vi "SANM_FreqMod_Host.vi"() -> ()   [LabVIEW 2012]
uses:
  <vilib>/FPGAPlugInAG/PCI-7831R/niLvFpga_Open_PCI-7831R.vi
  <vilib>/Utility/error.llb/Error Cluster From Error Code.vi
  <vilib>/rvi/errors/niLvFpgaAdjustHostInterfaceError.vi
  <vilib>/FPGAPlugInAG/PCI-7831R/niLvFpga_Abort_PCI-7831R.vi
  <vilib>/FPGAPlugInAG/PCI-7831R/niLvFpga_Close_PCI-7831R.vi
  <vilib>/rvi/interface/nirviOpenFPGA/nirviOpenFPGA.xnode
  SB130-XPS/Documents/FPGA-project-apporach-retraction/FPGA Bitfiles/Apporach-Retract_FPGATarget2_SANMFreqMod-1a_mUEf4QzcPK8.lvbitx
  SANM_FreqMod-1a.vi
  <vilib>/rvi/interface/nirviReadWriteControl/nirviReadWriteControl.xnode
  <vilib>/rvi/interface/nirviMethod/nirviMethod.xnode
  <vilib>/rvi/interface/nirviCloseFPGA/nirviCloseFPGA.xnode
  NiFpgaLv.dll
panel:
  in  "millisecond multiple":u32=75
  out "Indicator":dbl=0.15
  in  "Sampling Frequency 2":i32=200000
  in  "PLL Input\nNominal \nFrequency":i32=30000
  out "R Graph":dbl(graph)
  out "Degree":dbl
  out "Y":dbl
  out "X":dbl
  out "F Graph":dbl(graph)
  in  "Sampling Frequency":dbl=200000.0
  out "Decimation":i32=977
  out "Stages":i32=1
  out "Dec2":i32=128
  out "Dec1":i32=1
  in  "Filter Rolloff":enum16{"20 dB", "40 dB", "60 dB", "80 dB"}(ring)
  in  "Time Constant [s]":dbl=2.5 min=0.0 step=0.0001 format="%.2f"
  in  "stop 2":bool
  in  "stop":bool
  out "K Indicator":dbl=1.52588e-05
  out "Nominal Freq Indicator":dbl=0.494873
  in  "K":dbl=1.52588e-05
  in  "Nominal Freq":dbl=0.494873
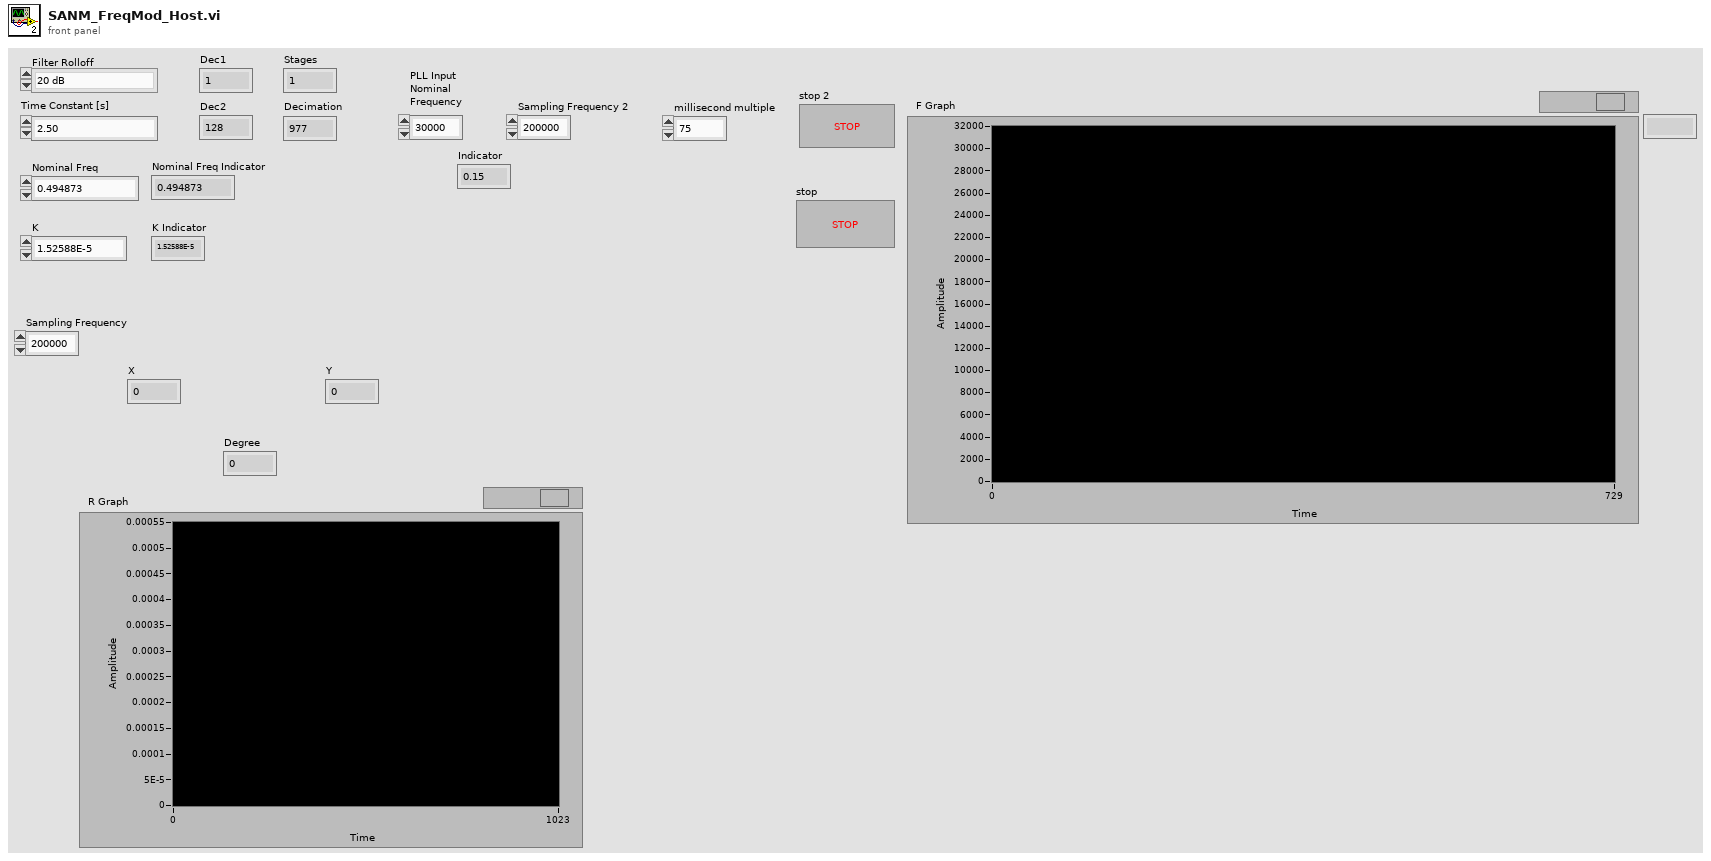
[diagram p1: front panel]
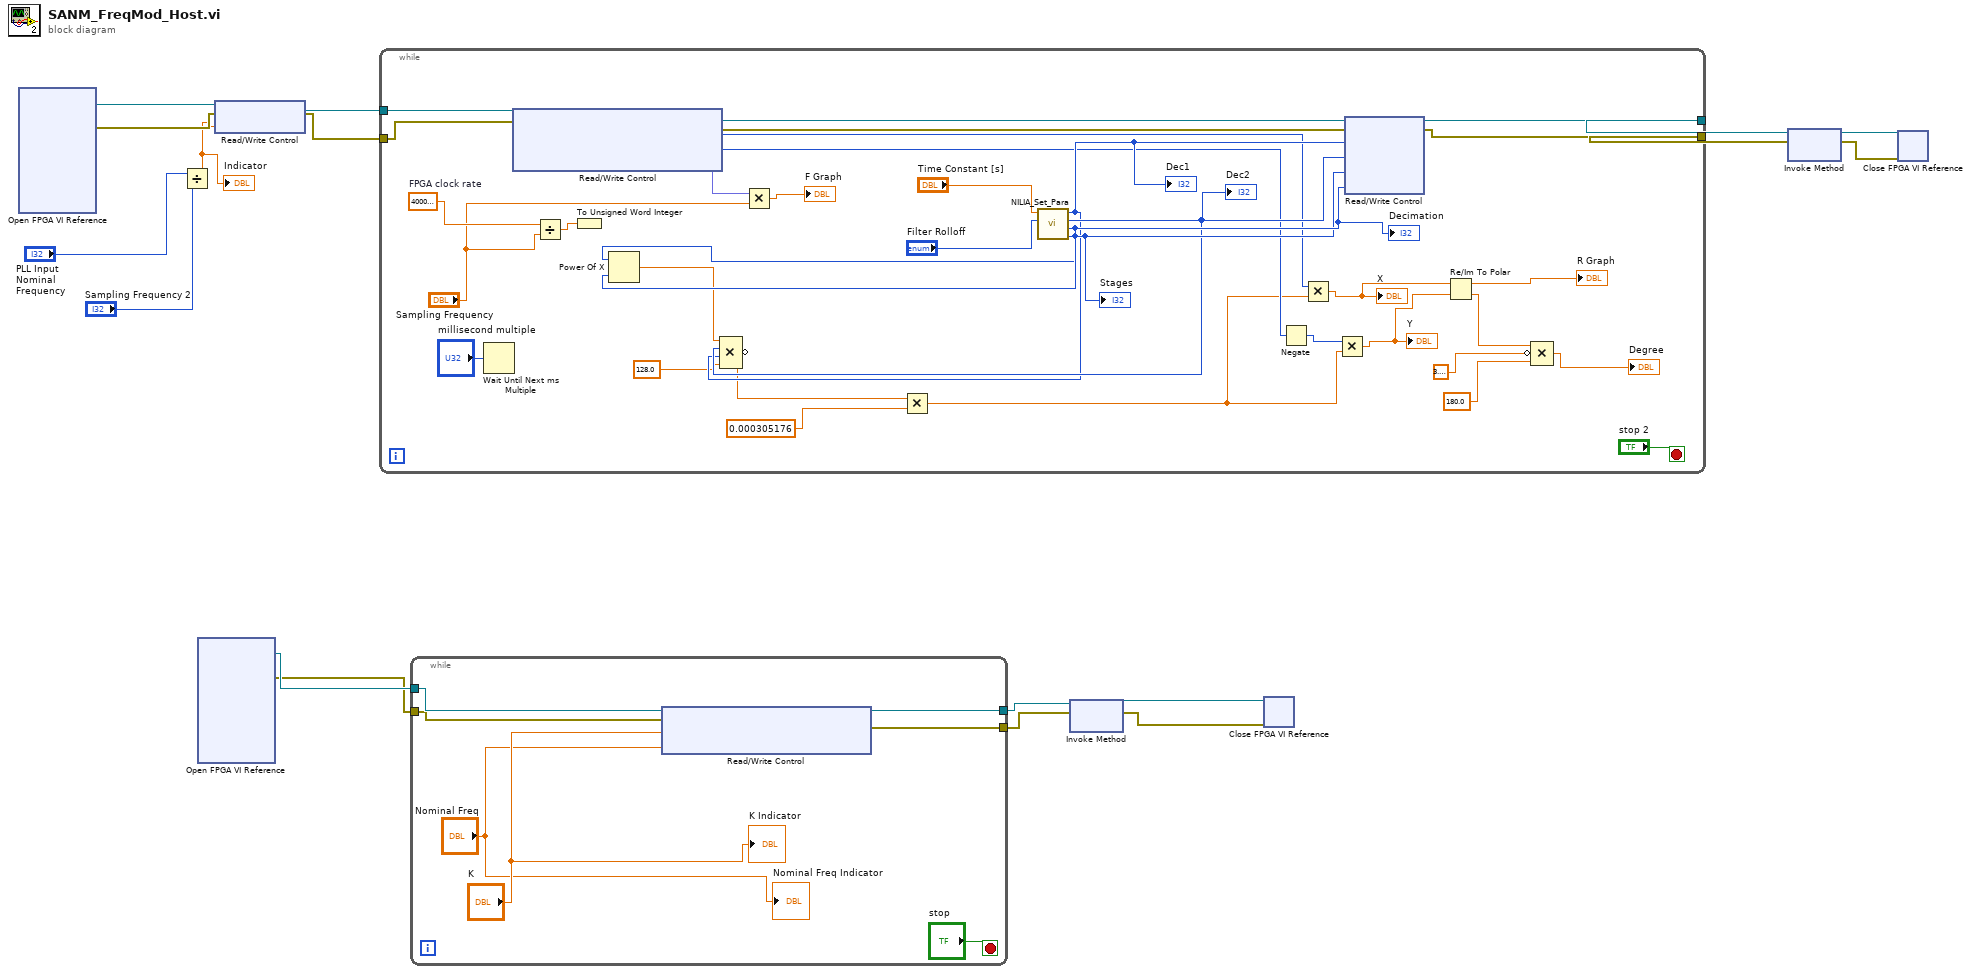
[diagram p0: block diagram]
diagram:
  n1 = xnode "Open FPGA VI Reference"() -> ("FPGA VI Reference Out"=w5:refnum<k20>, "error out"=w4:errorcluster)  [unwired: 2 in]
  n2 = Divide(x="PLL Input\nNominal \nFrequency", y="Sampling Frequency 2") -> (x/y=w1:dbl)
  "Indicator" <- w1
  n3 = xnode "Open FPGA VI Reference"() -> ("FPGA VI Reference Out"=w17:refnum<k20>, "error out"=w16:errorcluster)  [unwired: 2 in]
  n4 = xnode "Read/Write Control"("FPGA VI Reference In"=w5, "error in"=w4, "Nominal Freq"=w1) -> ("FPGA VI Reference Out"=w7:refnum<k20>, "error out"=w6:errorcluster)
  n5 = while {
    tunnel: w7 -> [w51]
    tunnel: w6 -> [w50]
    tunnel: [w47] -> w11
    tunnel: [w46] -> w10
    stop <- "stop 2" stop-if-true
    w21 = 40000000.0  # FPGA clock rate
    n6 = Wait Until Next ms Multiple(millisecond multiple="millisecond multiple") -> ()  [unwired: 1 out]
    n7 = xnode "Read/Write Control"("FPGA VI Reference In"=w51, "error in"=w50) -> ("FPGA VI Reference Out"=w49:refnum<k20>, "error out"=w48:errorcluster, "ChannelI"=w30:i64, "ChannelQ"=w31:i64, "f"=w33:fxp<+/-,32,0>)
    n8 = Divide(x=w21, y="Sampling Frequency") -> (x/y=w19:dbl)
    n9 = To Unsigned Word Integer(number=w19) -> ()  [unwired: 1 out]
    n10 = Multiply(x=w33, y="Sampling Frequency") -> (x*y=→"F Graph":dbl)
    n11 = call "NILIA_Set_Para.vi"("rolloff"="Filter Rolloff", "TC [sec]"="Time Constant [s]") -> ("3rd stages"=w41:i32, "3rd decimation"=w42:i32, "2nd decimation"=w39:i32, "1st decimation"=w38:i32)  [unwired: 5 in, 1 out]
    "Dec1" <- w38
    "Dec2" <- w39
    "Stages" <- w41
    "Decimation" <- w42
    n12 = Power Of X(1:w42, 2:w41) -> (0:w40:dbl)
    n13 = Compound Arithmetic op=MULTIPLY(w40, w39, w38, 128.0) -> (invert w36:dbl)
    n14 = Multiply(x=w36, y=0.000305176) -> (x*y=w29:dbl)
    n15 = Negate(x=w31) -> (-x=w32:i64)
    n16 = Multiply(x=w30, y=w29) -> (x*y=w25:dbl)
    "X" <- w25
    n17 = Multiply(x=w32, y=w29) -> (x*y=w26:dbl)
    "Y" <- w26
    n18 = xnode "Read/Write Control"("FPGA VI Reference In"=w49, "error in"=w48, "Dec1"=w38, "Dec2"=w39, "Stages"=w41, "Decimation"=w42) -> ("FPGA VI Reference Out"=w47:refnum<k20>, "error out"=w46:errorcluster)
    n19 = Re/Im To Polar(2:w26, 3:w25) -> (0:w27:dbl, 1:→"R Graph":dbl)
    n20 = Compound Arithmetic op=MULTIPLY(w27, invert 3.141592653589793, 180.0 ("value")) -> (→"Degree":dbl)
  }
  n21 = while {
    tunnel: w17 -> [w58]
    tunnel: w16 -> [w57]
    tunnel: [w56] -> w15
    tunnel: [w55] -> w14
    stop <- "stop" stop-if-true
    n22 = xnode "Read/Write Control"("FPGA VI Reference In"=w58, "error in"=w57, "K"="K", "Nominal Freq"="Nominal Freq") -> ("FPGA VI Reference Out"=w56:refnum<k20>, "error out"=w55:errorcluster)
    "Nominal Freq Indicator" <- "Nominal Freq"
    "K Indicator" <- "K"
  }
  n23 = xnode "Invoke Method"("FPGA VI Reference In"=w15, "error in"=w14) -> ("FPGA VI Reference Out"=w13:refnum<k20>, "error out"=w12:errorcluster)
  n24 = xnode "Close FPGA VI Reference"("FPGA VI Reference In"=w13, "error in"=w12) -> ()  [unwired: 1 out]
  n25 = xnode "Invoke Method"("FPGA VI Reference In"=w11, "error in"=w10) -> ("FPGA VI Reference Out"=w9:refnum<k20>, "error out"=w8:errorcluster)
  n26 = xnode "Close FPGA VI Reference"("FPGA VI Reference In"=w9, "error in"=w8) -> ()  [unwired: 1 out]
